vi "SeCrTs-Continuous or cummulative.vi"(8 "AI  data":dbl[](array[numeric]), 9 "AI Channels Name LP":string[](array[string]), 10 "CDT":dbl, 11 "output cluster":T1) -> (2 "Failure case Seq":string, 3 "In Range":string)   [LabVIEW 2022 SP3]
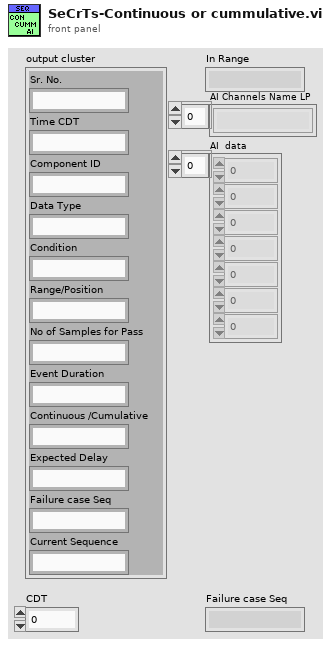
[diagram p1: front panel]
types:
  T1 = cluster{"Sr. No.":string, "Time CDT":string, "Component ID":string, "Data Type":string, "Condition":string, "Range/Position":string, "No of Samples for Pass":string, "Event Duration":string, "Continuous /Cumulative":string, "Expected Delay":string, "Failure case Seq":string, "Current Sequence":string}
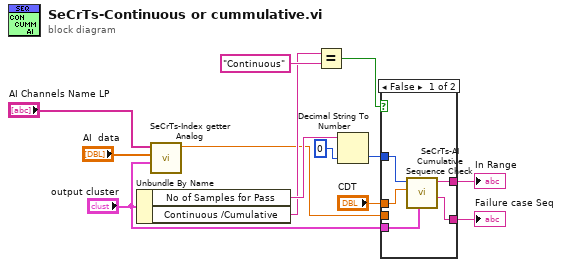
[diagram p0: block diagram]
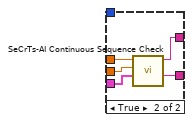
[diagram p2: hidden frame]
diagram:
  n1 = Unbundle By Name("output cluster") -> ("No of Samples for Pass"=w9:string, "Continuous /Cumulative"=w5:string)
  n2 = call "SeCrTs-Index getter Analog.vi"("output cluster"="output cluster", "AI Y  data"="AI  data", "AI Channels Name"="AI Channels Name LP") -> ("Analog data"=w4:dbl)  [unwired: 8 in]
  n3 = Equal?(x=w5, y="Continuous") -> (x = y?=w7:bool)
  n4 = Decimal String To Number(string=w9, default (0L)=0) -> (number=w10:i32)  [unwired: 1 in, 1 out]
  n5 = case shown="False" w7 {
    tunnel: w4 -> [_ w19]
    tunnel: "output cluster" -> [w16 w20]
    tunnel: w10 -> [w18 _]
    tunnel: [w15 w23] -> w13
    tunnel: [w14 w22] -> w12
    tunnel: "CDT" -> [w17 w21]
    frame False {
      n6 = call "SeCrTs-AI Cumulative Sequence Check.vi"("output cluster"=w16, "CDT"=w17, "Loop no"=w18) -> ("Failure case Seq"=w14:string, "String"=w15:string)  [unwired: 5 in, 1 out]
    }
    frame True {
      n7 = call "SeCrTs-AI Continuous Sequence Check.vi"("output cluster"=w20, "AI"=w19, "CDT"=w21) -> ("Failure case Seq"=w22:string, "In Range"=w23:string)  [unwired: 6 in, 1 out]
    }
  }
  "In Range" <- w13
  "Failure case Seq" <- w12
